vi "Save data file (pass-fail) v5.vi"(8 "Input Cluster":T1, 11 "panel id":string) -> (0 "network file save error":errorcluster, 3 "file save path":string)   [LabVIEW 2013]
uses:
  program files/Global 1.vi
panel:
  out "status":string
  out "C drive root path":string
  out "network file dir path":path
  out "network dir":string
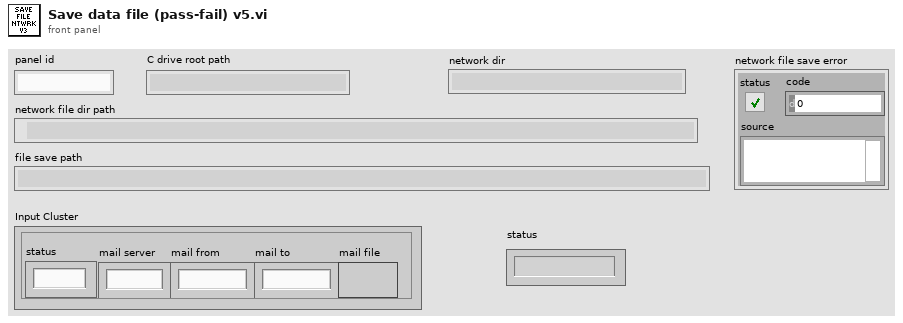
[diagram p1: front panel]
types:
  T1 = cluster{"status":string, "mail server":string, "mail from":string, "mail to":string, "mail file":bool}
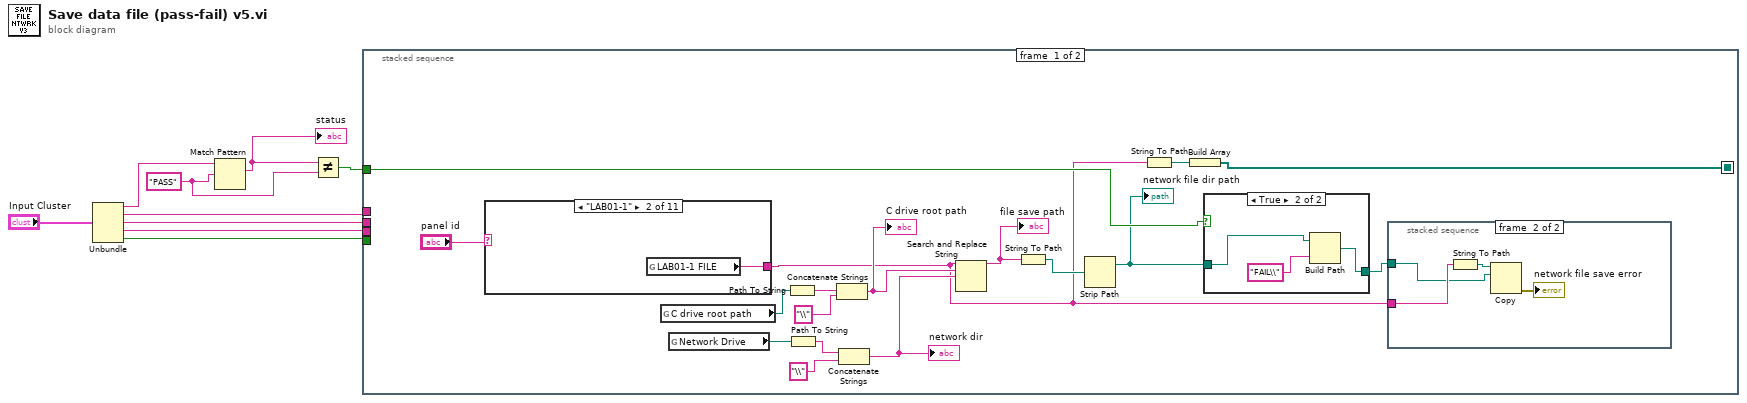
[diagram p0: block diagram]
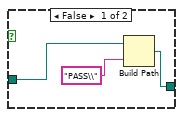
[diagram p2: hidden frame]
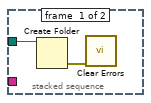
[diagram p3: hidden frame]
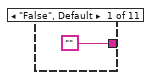
[diagram p4: hidden frame]
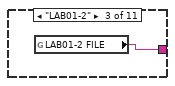
[diagram p5: hidden frame]
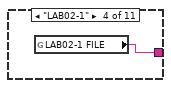
[diagram p6: hidden frame]
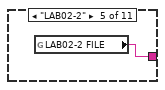
[diagram p7: hidden frame]
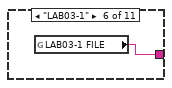
[diagram p8: hidden frame]
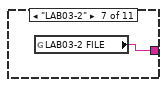
[diagram p9: hidden frame]
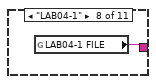
[diagram p10: hidden frame]
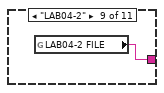
[diagram p11: hidden frame]
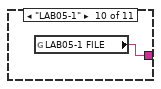
[diagram p12: hidden frame]
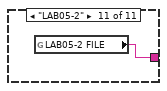
[diagram p13: hidden frame]
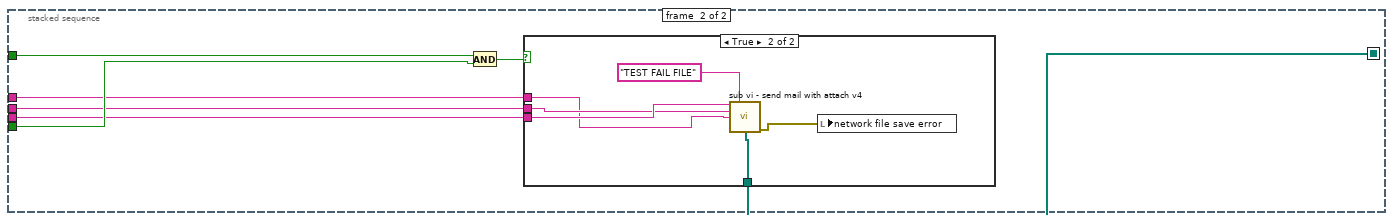
[diagram p14: hidden frame]
diagram:
  w9 = "PASS"
  n1 = Unbundle("Input Cluster") -> ("status"=w7:string, "mail server"=w1:string, "mail from"=w2:string, "mail to"=w3:string, "mail file"=w4:bool)
  n2 = Match Pattern(string=w7, regular expression=w9) -> (match substring=w8:string)  [unwired: 1 in, 3 out]
  "status" <- w8
  n3 = Not Equal?(x=w8, y=w9) -> (x != y?=w5:bool)
  n4 = stacked-sequence {
    seq-local: [w15 _] -> [_ w55]
    tunnel: w5 -> [w14 w54]
    tunnel: w4 -> [_ w53]
    tunnel: w3 -> [_ w52]
    tunnel: w2 -> [_ w51]
    tunnel: w1 -> [_ w50]
    frame #0 {
      n5 = case shown="\"LAB01-1\"" "panel id" {
        tunnel: ["" w40 w41 w42 w43 w44 w45 w46 w47 w48 w49] -> w10
        frame "False", Default {
        }
        frame "LAB01-1" {
          n6 = global read "Global 1.vi" "LAB01-1 FILE"() -> (w40:string)
        }
        frame "LAB01-2" {
          n7 = global read "Global 1.vi" "LAB01-2 FILE"() -> (w41:string)
        }
        frame "LAB02-1" {
          n8 = global read "Global 1.vi" "LAB02-1 FILE"() -> (w42:string)
        }
        frame "LAB02-2" {
          n9 = global read "Global 1.vi" "LAB02-2 FILE"() -> (w43:string)
        }
        frame "LAB03-1" {
          n10 = global read "Global 1.vi" "LAB03-1 FILE"() -> (w44:string)
        }
        frame "LAB03-2" {
          n11 = global read "Global 1.vi" "LAB03-2 FILE"() -> (w45:string)
        }
        frame "LAB04-1" {
          n12 = global read "Global 1.vi" "LAB04-1 FILE"() -> (w46:string)
        }
        frame "LAB04-2" {
          n13 = global read "Global 1.vi" "LAB04-2 FILE"() -> (w47:string)
        }
        frame "LAB05-1" {
          n14 = global read "Global 1.vi" "LAB05-1 FILE"() -> (w48:string)
        }
        frame "LAB05-2" {
          n15 = global read "Global 1.vi" "LAB05-2 FILE"() -> (w49:string)
        }
      }
      n16 = global read "Global 1.vi" "C drive root path"() -> (w18:path)
      n17 = global read "Global 1.vi" "Network Drive"() -> (w25:path)
      n18 = Path To String(path=w18) -> (string=w19:string)
      n19 = Path To String(path=w25) -> (string=w24:string)
      n20 = Concatenate Strings(w19, "\\") -> (w17:string)
      "C drive root path" <- w17
      n21 = Concatenate Strings(w24, "\\") -> (w22:string)
      "network dir" <- w22
      n22 = Search and Replace String(input string=w10, search string=w17, replace string=w22) -> (result string=w21:string)  [unwired: 5 in, 3 out]
      "file save path" <- w21
      n23 = String To Path(string=w21) -> (path=w16:path)
      n24 = Strip Path(path=w16) -> (stripped path=w12:path)  [unwired: 1 out]
      "network file dir path" <- w12
      n25 = String To Path(string=w10) -> (path=w11:path)
      n26 = Build Array(w11) -> (w15:path[])
      n27 = case shown="True" w14 {
        tunnel: [w27 w32] -> w13
        tunnel: w12 -> [w28 w30]
        frame False {
          n28 = Build Path(base path=w28, name or relative path="PASS\\") -> (appended path=w27:path)
        }
        frame True {
          n29 = Build Path(base path=w30, name or relative path="FAIL\\") -> (appended path=w32:path)
        }
      }
      n30 = stacked-sequence {
        tunnel: w13 -> [w34 w35]
        tunnel: w10 -> [_ w36]
        frame #0 {
          n31 = Create Folder(path (use dialog)=w34) -> (error out=w33:errorcluster)  [unwired: 2 in, 2 out]
          n32 = call <vilib>:"Clear Errors.vi"("error in (no error)"=w33) -> ()  [unwired: 6 in, 1 out]
        }
        frame #1 {
          n33 = String To Path(string=w36) -> (path=w37:path)
          n34 = Copy(10:w35, 11:w37) -> (0:→"network file save error":errorcluster)  [unwired: 3 in, 2 out]
        }
      }
    }
    frame #1 {
      n35 = And(x=w54, y=w53) -> (x .and. y?=w56:bool)
      n36 = case shown="True" w56 {
        tunnel: w55 -> [_ w61]
        tunnel: w52 -> [_ w59]
        tunnel: w51 -> [_ w58]
        tunnel: w50 -> [_ w57]
        frame False {
        }
        frame True {
          n37 = call "sub vi - send mail with attach v4.vi"("TO:"=w59, "subject"="TEST FAIL FILE", "from"=w58, "out going server"=w57, "Attachements"=w61) -> ("error out"=w62:errorcluster)  [unwired: 10 in]
          n38 = local write "network file save error"(w62) -> ()
        }
      }
    }
  }
